vi "mainSMS.vi"() -> ()   [LabVIEW 2012]
uses:
  <vilib>/Platform/TimedLoop/XDataNode/timing_clust.ctl
  <vilib>/Platform/TimedLoop/XDataNode/nitl_modes.ctl
  <vilib>/Platform/TimedLoop/XDataNode/wakeup.ctl
  <vilib>/platform/TimedLoop/XDataNode/XDataNode.xnode
  <vilib>/Platform/TimedLoop/XDataNode/XDNodeRunTimeDep.lvlib
panel:
  in  "num":string
  in  "sms":string
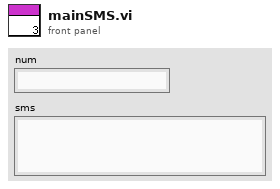
[diagram p1: front panel]
types:
  T1 = typedef "XDNodeRunTimeDep.lvlib/timing_clust.ctl" = cluster{"Expected End [f-1]":u64, "Actual End [f-1]":u64, "Finished Late? [f-1]":bool, "Expected End [i-1]":u64, "Actual End [i-1]":u64, "Finished Late? [i-1]":bool, "Expected Start [i]":u64, "Actual Start [i]":u64, "Expected Start [f]":u64, "Actual Start [f]":u64, "Source Name":string, "Structure Name":string, "Period":i64, "Deadline":i64, "Offset":i64, "Start":i64, "Priority":i32, "Timeout":i32, "Mode":T2, "Wakeup Reason":T3, "Error":errorcluster, "Source Type":string, "Secondary Source Type":string, "Global End Time":u64, "Global Start Time":u64, "Frame Duration":u64, "Iteration Duration":u64, "Assigned CPU":i32, "I/O Scan Engine Mode":u32}
  T2 = typedef "XDNodeRunTimeDep.lvlib/nitl_modes.ctl" = enum32{"No Change", "Process missed periods, maintain original phase", "Discard missed periods, maintain original phase", "Process missed periods, ignore original phase", "Discard missed periods, ignore original phase"}
  T3 = typedef "XDNodeRunTimeDep.lvlib/wakeup.ctl" = enum32{"Normal", "Aborted", "Asynchronous wakeup", "Timing source error", "Timed loop error", "Timeout"}
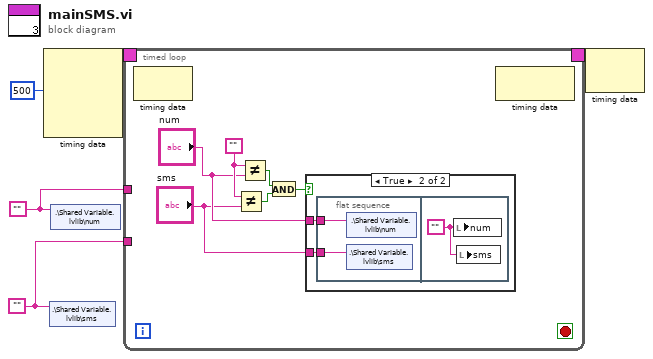
[diagram p0: block diagram]
diagram:
  w1 = ""
  w2 = ""
  n1 = node-c288(i64 500 ("Period")) -> (w5:T1)  [unwired: 3 in]
  n2 = shared-variable ".\\Shared Variable.lvlib\\sms"(w1) -> ()  [unwired: 1 in, 1 out]
  n3 = shared-variable ".\\Shared Variable.lvlib\\num"(w2) -> ()  [unwired: 1 in, 1 out]
  n4 = timed-loop {
    timing: w5 -> [_]
    timing-out: [_] -> w4
    tunnel: w2 -> [_]
    tunnel: w1 -> [_]
    stop <- _ stop-if-true
    w11 = ""
    n5 = node-c288() -> ()  [unwired: 1 in, 1 out]
    n6 = Not Equal?(x=w11, y="sms") -> (x != y?=w10:bool)
    n7 = Not Equal?(x=w11, y="num") -> (x != y?=w9:bool)
    n8 = And(x=w9, y=w10) -> (x .and. y?=w8:bool)
    n9 = case shown="True" w8 {
      tunnel: "num" -> [_ w13]
      tunnel: "sms" -> [_ w12]
      frame False {
      }
      frame True {
        n10 = flat-sequence {
          tunnel: w13 -> [w15]
          tunnel: w12 -> [w14]
          frame #0 {
            n11 = shared-variable ".\\Shared Variable.lvlib\\num"(w15) -> ()  [unwired: 1 in, 1 out]
            n12 = shared-variable ".\\Shared Variable.lvlib\\sms"(w14) -> ()  [unwired: 1 in, 1 out]
          }
          frame #1 {
            w16 = ""
            n13 = local write "num"(w16) -> ()
            n14 = local write "sms"(w16) -> ()
          }
        }
      }
    }
    n15 = node-c288() -> ()  [unwired: 1 in, 1 out]
  }
  n16 = node-c288(w4) -> ()  [unwired: 1 out]
